vi "Process.vi"(11 "Actor":refnum<class "Task Scheduler Actor.lvclass">) -> ()   [LabVIEW 2021, in "Task Scheduler Actor.lvclass"]
uses:
  Task Scheduler Actor.lvclass
  Task Scheduler Actor.lvclass/Task Scheduler Actor.ctl
  <vilib>/platform/TimedLoop/XDataNode/XDataNode.xnode
  Re-use Libraries/Minimal Actor Framework/Actors/Base Actor/Actor/Front Panel State.ctl
  Re-use Libraries/Minimal Actor Framework/Actors/Base Actor/Actor/Actor.lvclass
  Re-use Libraries/Minimal Actor Framework/Messaging/Message/Message.lvclass
  Error Handler/API/Error Handler Actor API.lvclass
  Re-use Libraries/Timer/Timer.lvclass
  Timer Config.ctl
  <vilib>/Platform/TimedLoop/XDataNode/nitl_modes.ctl
  <vilib>/Platform/TimedLoop/XDataNode/XDNodeRunTimeDep.lvlib
  <vilib>/Platform/TimedLoop/XDataNode/wakeup.ctl
  <vilib>/Platform/TimedLoop/XDataNode/timing_clust.ctl
  <vilib>/Utility/miscctls.llb/LVRowAndColumnTypeDef.ctl
  Main Controller/API/Main Controller Actor API.lvclass
panel:
  out "Tasks":string[][](table)
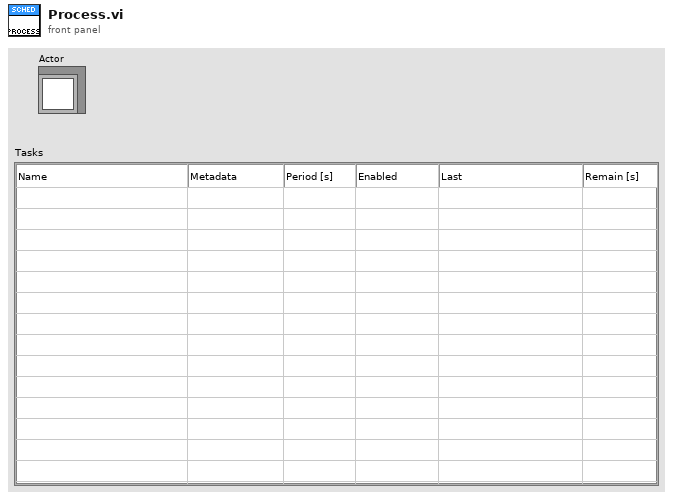
[diagram p1: front panel]
types:
  T1 = typedef "LVRowAndColumnTypeDef.ctl" = cluster{"Row":i32, "Column":i32}
  T2 = typedef "XDNodeRunTimeDep.lvlib/timing_clust.ctl" = cluster{"Expected End [f-1]":u64, "Actual End [f-1]":u64, "Finished Late? [f-1]":bool, "Expected End [i-1]":u64, "Actual End [i-1]":u64, "Finished Late? [i-1]":bool, "Expected Start [i]":u64, "Actual Start [i]":u64, "Expected Start [f]":u64, "Actual Start [f]":u64, "Source Name":string, "Structure Name":string, "Period":i64, "Deadline":i64, "Offset":i64, "Start":i64, "Priority":i32, "Timeout":i32, "Mode":T3, "Wakeup Reason":T4, "Error":errorcluster, "Source Type":string, "Secondary Source Type":string, "Global End Time":u64, "Global Start Time":u64, "Frame Duration":u64, "Iteration Duration":u64, "Assigned CPU":i32, "I/O Scan Engine Mode":u32}
  T3 = typedef "XDNodeRunTimeDep.lvlib/nitl_modes.ctl" = enum32{"No Change", "Process missed periods, maintain original phase", "Discard missed periods, maintain original phase", "Process missed periods, ignore original phase", "Discard missed periods, ignore original phase"}
  T4 = typedef "XDNodeRunTimeDep.lvlib/wakeup.ctl" = enum32{"Normal", "Aborted", "Asynchronous wakeup", "Timing source error", "Timed loop error", "Timeout"}
  T5 = typedef "Actor.lvclass/Front Panel State.ctl" = enum32{"Invalid", "Standard", "Closed", "Hidden", "Minimized", "Maximized"}
  T6 = typedef "Task Scheduler Actor.lvclass/Timer Config.ctl" = cluster{"Name":string, "Period [s]":dbl, "Enabled":bool, "Metadata":string}
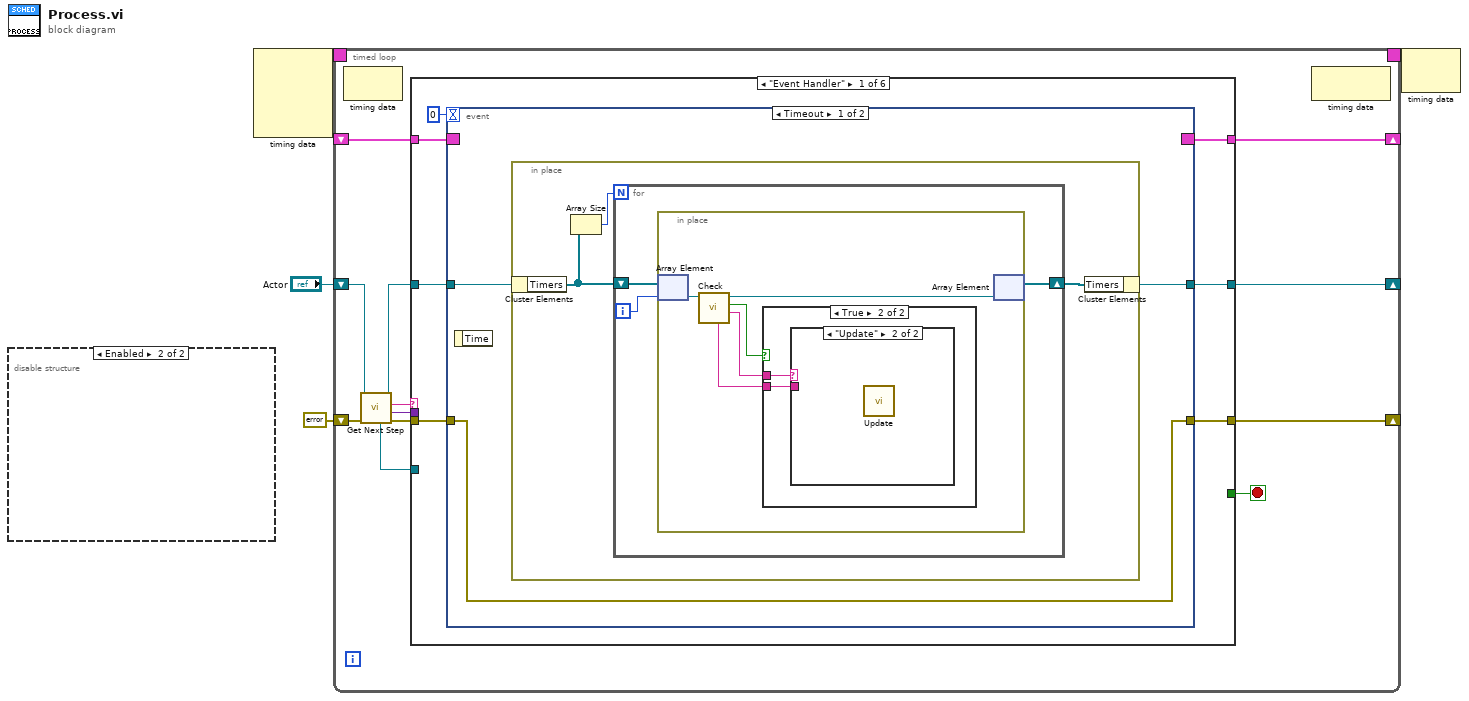
[diagram p0: block diagram]
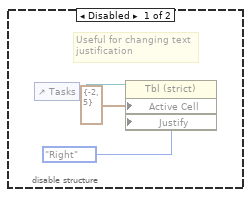
[diagram p2: hidden frame]
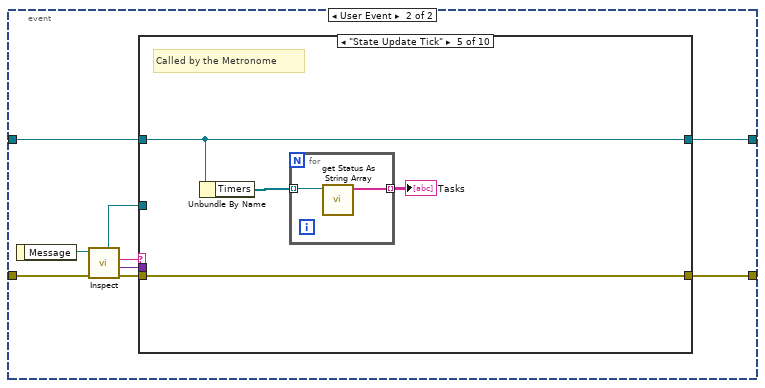
[diagram p5: hidden frame]
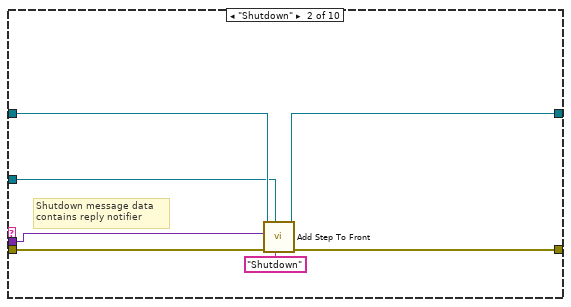
[diagram p7: hidden frame]
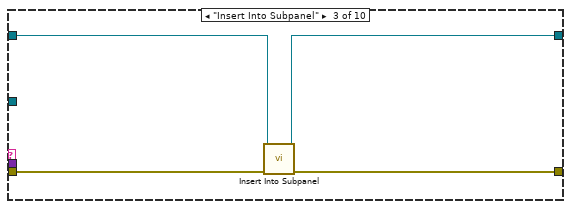
[diagram p8: hidden frame]
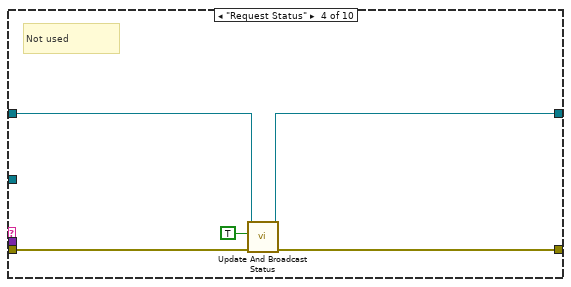
[diagram p9: hidden frame]
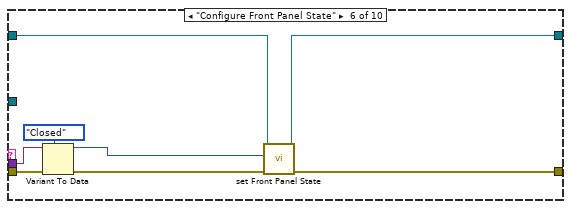
[diagram p10: hidden frame]
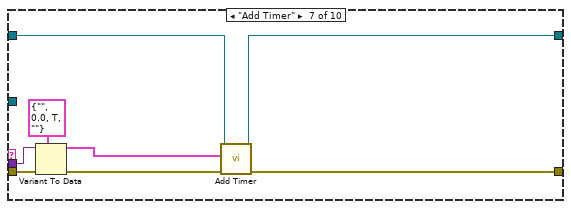
[diagram p11: hidden frame]
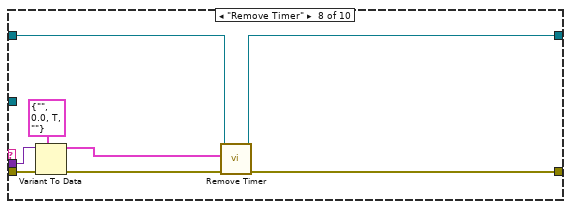
[diagram p12: hidden frame]
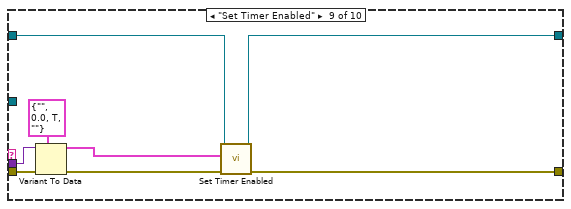
[diagram p13: hidden frame]
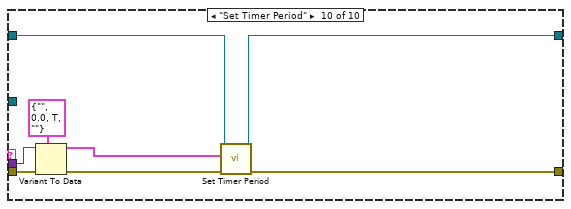
[diagram p14: hidden frame]
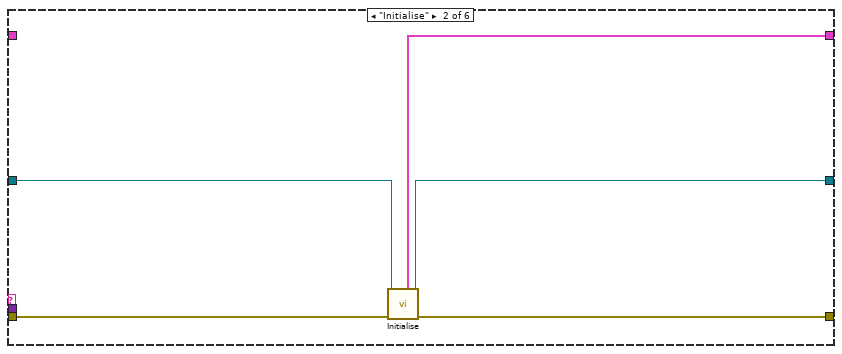
[diagram p15: hidden frame]
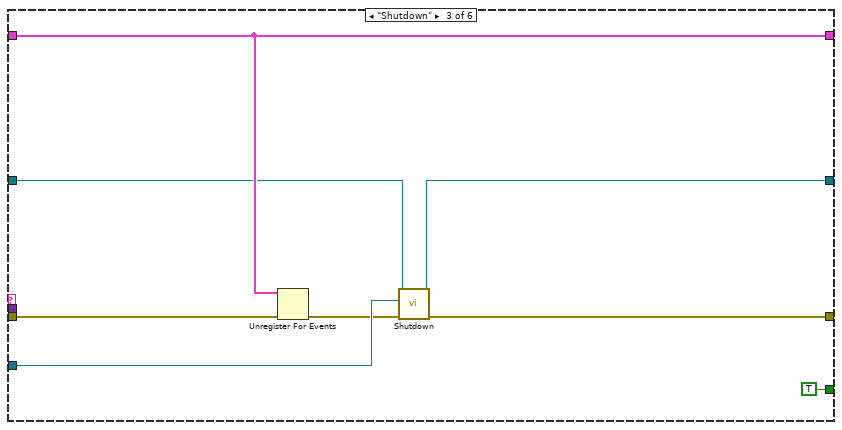
[diagram p16: hidden frame]
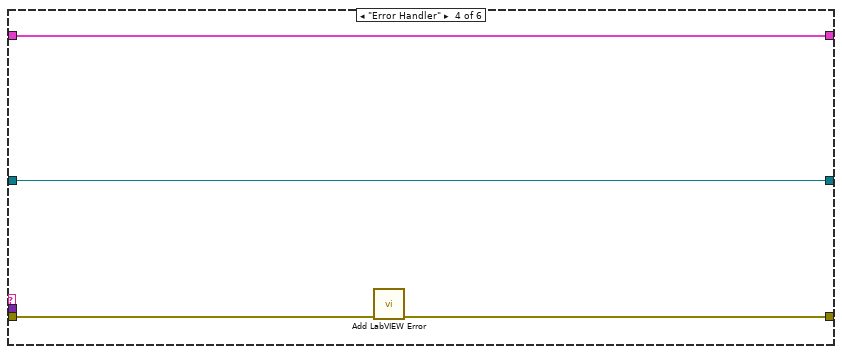
[diagram p17: hidden frame]
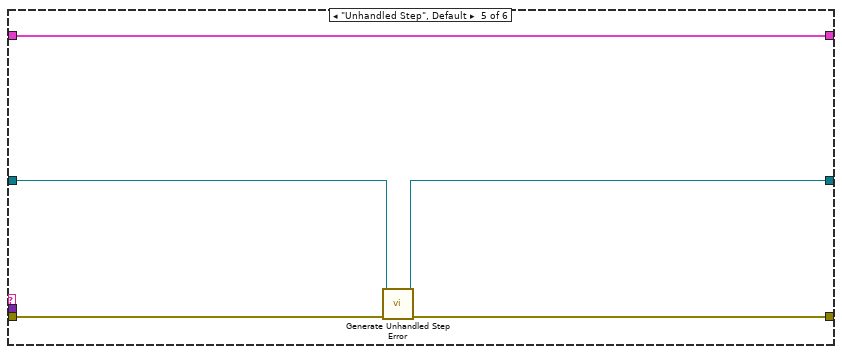
[diagram p18: hidden frame]
diagram:
  n1 = disable-structure shown="Enabled" {
    frame Disabled {
      # "Useful for changing text justification"
      n2 = control-ref of="Tasks"() -> (w7:refnum<vi>)
      n3 = property class="Tbl (strict)"(reference=w7, "Active Cell"=T1 {"Row"=-2, "Column"=5} ("Active Cell:Active Cell"), "Justify"=enum16{"Left", "Center", "Right"}."Right" ("Active Cell:Cell Justification")) -> ()  [unwired: 1 in, 2 out]
    }
    frame Enabled {
    }
  }
  n4 = node-c288() -> (w2:T2)  [unwired: 4 in]
  n5 = timed-loop {
    shift-right: [w10] -> _
    shift-left: "Actor" -> [w18]
    shift-right: [w15] -> _
    shift-left: _ -> [w14]
    shift-right: [w9] -> _
    shift-left: errorcluster {"status"=FALSE, "code"=0, "source"=""} ("error constant") -> [w12]
    timing: w2 -> [_]
    timing-out: [_] -> w1
    stop <- w19 stop-if-true
    n6 = node-c288() -> ()  [unwired: 1 in, 1 out]
    n7 = call-dynamic "Get Next Step.vi"("error in (no error)"=w12, "Actor in"=w18) -> ("error out"=w13:errorcluster, "Parameter"=w16:variant, "Step"=w11:string, "Actor out"=w17:refnum<class "Task Scheduler Actor.lvclass">, "Reply Channel"=w8:refnum<notifier>)  [unwired: 5 in]
    n8 = case shown="\"Event Handler\"" w11 {
      tunnel: [_ _ TRUE _ _ _] -> w19
      tunnel: w17 -> [w28 w122 w128 w133 w138 w141]
      tunnel: [w27 w120 w127 w133 w137 w141] -> w10
      tunnel: w16 -> [_ _ _ _ _ _]
      tunnel: [w25 w118 w129 w134 w139 w142] -> w15
      tunnel: w14 -> [w26 _ w129 w134 w139 w142]
      tunnel: w13 -> [w24 w121 w125 w132 w136 w140]
      tunnel: [w23 w119 w123 w131 w135 w140] -> w9
      tunnel: w8 -> [_ _ w126 _ _ _]
      frame "Event Handler" {
        n9 = event shown="[0] Timeout" {
          selector: w26 -> [_ _]
          dyn-events: [_ _] -> w25
          timeout: 0 -> [_ _]
          tunnel: w28 -> [w31 w53]
          tunnel: [w30 w52] -> w27
          tunnel: w24 -> [w29 w50]
          tunnel: [w29 w51] -> w23
          event Timeout {
            n10 = event-data() -> ()  [unwired: 1 in, 1 out]
            n11 = in-place {
              n12 = in-place-cluster #1(w31) -> ("Timers"=w33:refnum<class "Timer.lvclass">[])
              n13 = Array Size(array=w33) -> (size(s)=w32:i32)
              n14 = for {
                N: w32 -> [_]
                shift-right: [w35] -> w34
                shift-left: w33 -> [w37]
                i -> [w36]
                n15 = in-place {
                  n16 = in-place-array #2(w37, w36) -> (w42:refnum<class "Timer.lvclass">)
                  n17 = call "Check.vi"("Timer in"=w42) -> ("Name"=w40:string, "Elapsed"=w41:bool, "Timer out"=w39:refnum<class "Timer.lvclass">, "Metadata"=w38:string)  [unwired: 7 in]
                  n18 = case shown="True" w41 {
                    tunnel: w40 -> [_ w44]
                    tunnel: w38 -> [_ w43]
                    frame False {
                    }
                    frame True {
                      n19 = case shown="\"Update\"" w44 {
                        tunnel: w43 -> [_ _]
                        frame Default {
                        }
                        frame "Update" {
                          n20 = call "Update.vi"() -> ()  [unwired: 11 in, 1 out]
                        }
                      }
                    }
                  }
                  n21 = in-place-array #2(w39) -> (w35:refnum<class "Timer.lvclass">[])  [unwired: 1 out]
                }
              }
              n22 = in-place-cluster #1("Timers"=w34) -> (w30:refnum<class "Task Scheduler Actor.lvclass">)
            }
          }
          event User Event {
            n23 = event-data() -> ("Message"=w49:refnum<class "Message.lvclass">)  [unwired: 1 in]
            n24 = call "Inspect.vi"("error in (no error)"=w50, "Message in"=w49) -> ("error out"=w46:errorcluster, "Data"=w47:variant, "Name"=w48:string, "Reply Channel"=w45:refnum<notifier>)  [unwired: 5 in, 1 out]
            n25 = case shown="\"State Update Tick\"" w48 {
              tunnel: w53 -> [w55 w62 w66 w68 w75 w85 w93 w101 w109 w117]
              tunnel: [w55 w61 w65 w67 w75 w84 w92 w100 w108 w116] -> w52
              tunnel: w46 -> [w54 w59 w64 w70 w72 w81 w90 w98 w106 w114]
              tunnel: [w54 w58 w63 w69 w72 w83 w91 w99 w107 w115] -> w51
              tunnel: w47 -> [_ w57 _ _ _ w82 w89 w97 w105 w113]
              tunnel: w45 -> [_ w56 _ _ _ _ _ _ _ _]
              frame Default {
              }
              frame "Shutdown" {
                # "Shutdown message data contains reply notifier"
                n26 = call-dynamic "Add Step To Front.vi"("Step Name"="Shutdown", "Reply Channel"=w56, "error in (no error)"=w59, "Parameter"=w57, "Actor in"=w62) -> ("error out"=w58:errorcluster, "Actor out"=w61:refnum<class "Task Scheduler Actor.lvclass">)  [unwired: 5 in]
              }
              frame "Insert Into Subpanel" {
                n27 = call-dynamic "Insert Into Subpanel.vi"("error in (no error)"=w64, "Actor in"=w66) -> ("error out"=w63:errorcluster, "Actor out"=w65:refnum<class "Task Scheduler Actor.lvclass">)  [unwired: 8 in]
              }
              frame "Request Status" {
                # "Not used"
                n28 = call-dynamic "Update And Broadcast Status.vi"("error in (no error)"=w70, "OK"=TRUE, "Actor in"=w68) -> ("error out"=w69:errorcluster, "Actor out"=w67:refnum<class "Task Scheduler Actor.lvclass">)  [unwired: 7 in]
              }
              frame "State Update Tick" {
                # "Called by the Metronome"
                n29 = Unbundle By Name(w75) -> ("Timers"=w74:refnum<class "Timer.lvclass">[])
                n30 = for {
                  tunnel: w74 -> [w77] mode=indexing
                  tunnel: [w76] -> w73 mode=indexing
                  n31 = call "get Status As String Array.vi"("Timer in"=w77) -> ("Status"=w76:string[])  [unwired: 10 in]
                }
                "Tasks" <- w73
              }
              frame "Configure Front Panel State" {
                n32 = Variant To Data(error in=w81, type=Front_Panel_State."Closed" ("Front Panel State"), Variant=w82) -> (data=w78:T5, error out=w80:errorcluster)
                n33 = call-dynamic "set Front Panel State.vi"("error in (no error)"=w80, "Front Panel State"=w78, "Actor in"=w85) -> ("error out"=w83:errorcluster, "Actor out"=w84:refnum<class "Task Scheduler Actor.lvclass">)  [unwired: 7 in]
              }
              frame "Add Timer" {
                n34 = Variant To Data(error in=w90, type=T6 {"Name"="", "Period [s]"=0.0, "Enabled"=TRUE, "Metadata"=""} ("Timer Config"), Variant=w89) -> (data=w86:T6, error out=w87:errorcluster)
                n35 = call "Add Timer.vi"("error in (no error)"=w87, "Timer Config"=w86, "Task Scheduler Actor in"=w93) -> ("error out"=w91:errorcluster, "Task Scheduler Actor out"=w92:refnum<class "Task Scheduler Actor.lvclass">)  [unwired: 7 in]
              }
              frame "Remove Timer" {
                n36 = Variant To Data(error in=w98, type=T6 {"Name"="", "Period [s]"=0.0, "Enabled"=TRUE, "Metadata"=""} ("Timer Config"), Variant=w97) -> (data=w94:T6, error out=w95:errorcluster)
                n37 = call "Remove Timer.vi"("error in (no error)"=w95, "Timer Config"=w94, "Task Scheduler Actor in"=w101) -> ("error out"=w99:errorcluster, "Task Scheduler Actor out"=w100:refnum<class "Task Scheduler Actor.lvclass">)  [unwired: 7 in]
              }
              frame "Set Timer Enabled" {
                n38 = Variant To Data(error in=w106, type=T6 {"Name"="", "Period [s]"=0.0, "Enabled"=TRUE, "Metadata"=""} ("Timer Config"), Variant=w105) -> (data=w102:T6, error out=w103:errorcluster)
                n39 = call "Set Timer Enabled.vi"("error in (no error)"=w103, "Timer Config"=w102, "Timers Manager Actor in"=w109) -> ("error out"=w107:errorcluster, "Timers Manager Actor out"=w108:refnum<class "Task Scheduler Actor.lvclass">)  [unwired: 7 in]
              }
              frame "Set Timer Period" {
                n40 = Variant To Data(error in=w114, type=T6 {"Name"="", "Period [s]"=0.0, "Enabled"=TRUE, "Metadata"=""} ("Timer Config"), Variant=w113) -> (data=w110:T6, error out=w111:errorcluster)
                n41 = call "Set Timer Period.vi"("error in (no error)"=w111, "Timer Config"=w110, "Timers Manager Actor in"=w117) -> ("error out"=w115:errorcluster, "Timers Manager Actor out"=w116:refnum<class "Task Scheduler Actor.lvclass">)  [unwired: 7 in]
              }
            }
          }
        }
      }
      frame "Initialise" {
        n42 = call "Initialise.vi"("error in (no error)"=w121, "Actor in"=w122) -> ("error out"=w119:errorcluster, "Actor out"=w120:refnum<class "Task Scheduler Actor.lvclass">, "Observers"=w118:cluster{"Actor":refnum<event-registration>})  [unwired: 7 in]
      }
      frame "Shutdown" {
        n43 = Unregister For Events(event registration refnum=w129, error in=w125) -> (error out=w124:errorcluster)
        n44 = call-dynamic "Shutdown.vi"("error in (no error)"=w124, "Reply Channel"=w126, "Actor in"=w128) -> ("error out"=w123:errorcluster, "Actor out"=w127:refnum<class "Task Scheduler Actor.lvclass">)  [unwired: 7 in]
      }
      frame "Error Handler" {
        n45 = call "Add LabVIEW Error.vi"("error in (no error)"=w132) -> ("error out"=w131:errorcluster)  [unwired: 10 in]
      }
      frame "Unhandled Step", Default {
        n46 = call-dynamic "Generate Unhandled Step Error.vi"("error in (no error)"=w136, "Actor in"=w138) -> ("error out"=w135:errorcluster, "Actor out"=w137:refnum<class "Task Scheduler Actor.lvclass">)  [unwired: 8 in]
      }
      frame "-----------------------" {
        # "Separator"
      }
    }
    n47 = node-c288() -> ()  [unwired: 1 in, 1 out]
  }
  n48 = node-c288(w1) -> ()  [unwired: 1 out]
